vi "Z900_navX_I2C_Read.vi"(8 "error in (no error)":errorcluster, 10 "Registry":u8[](array[numeric]), 11 "Interface TypeDefs":T1 {"I2CDevRef"."Device Address" format="%.0x"}) -> (0 "error out":errorcluster, 1 "Valid":bool, 2 "Registry":u8[](array[numeric]), 3 "Interface TypeDefs":T1 {"I2CDevRef"."Device Address" format="%.0x"})   [LabVIEW 2015, in "navX Library v2.lvlib"]
uses:
  navX Library v2.lvlib
  TypeDefs/Z900_navX_InterfaceTypeDef.ctl
  <vilib>/Rock Robotics/WPI/SerialPort/WPI_SerialPortRef.ctl
  <vilib>/Rock Robotics/WPI/I2C/WPI_I2CDevRef.ctl
  <vilib>/Rock Robotics/SystemInterfaces/i2clib/i2c_bus.ctl
  <vilib>/Rock Robotics/WPI/SPI/WPI_SPIDevRef.ctl
  <vilib>/Rock Robotics/SystemInterfaces/spilib/spi_bus.ctl
  TypeDefs/Z900_navX_DeviceRegisters.ctl
  TypeDefs/Flags/Z900_navX_Flags_CapabilityTypeDef.ctl
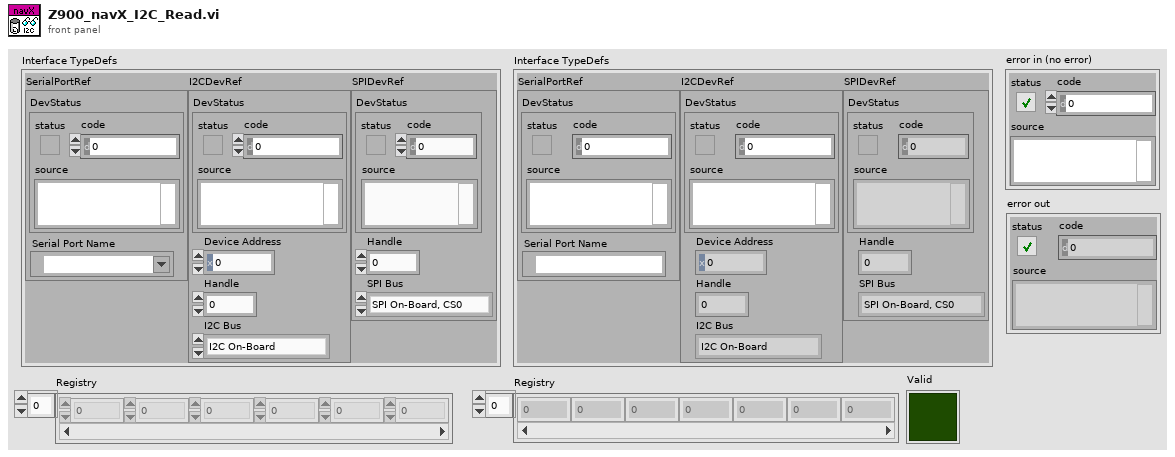
[diagram p1: front panel]
types:
  T1 = typedef "navX Library v2.lvlib/Z900_navX_InterfaceTypeDef.ctl" = cluster{"SerialPortRef":T2, "I2CDevRef":T3, "SPIDevRef":T5}
  T2 = typedef "WPI_SerialPortRef.ctl" = cluster{"DevStatus":errorcluster, "Serial Port Name":refnum<visa-resource-name>}
  T3 = typedef "WPI_I2CDevRef.ctl" = cluster{"DevStatus":errorcluster, "Device Address":u8, "Handle":i32, "I2C Bus":T4}
  T4 = typedef "i2c_bus.ctl" = enum16{"I2C On-Board", "I2C MXP", "Invalid"}
  T5 = typedef "WPI_SPIDevRef.ctl" = cluster{"DevStatus":errorcluster, "Handle":i32, "SPI Bus":T6}
  T6 = typedef "spi_bus.ctl" = enum16{"SPI On-Board, CS0", "SPI On-Board, CS1", "SPI On-Board, CS2", "SPI On-Board, CS3", "SPI MXP", "Invalid"}
  T7 = typedef "navX Library v2.lvlib/Z900_navX_DeviceRegisters.ctl" = u8
  T8 = typedef "navX Library v2.lvlib/Z900_navX_Flags_CapabilityTypeDef.ctl" = u16
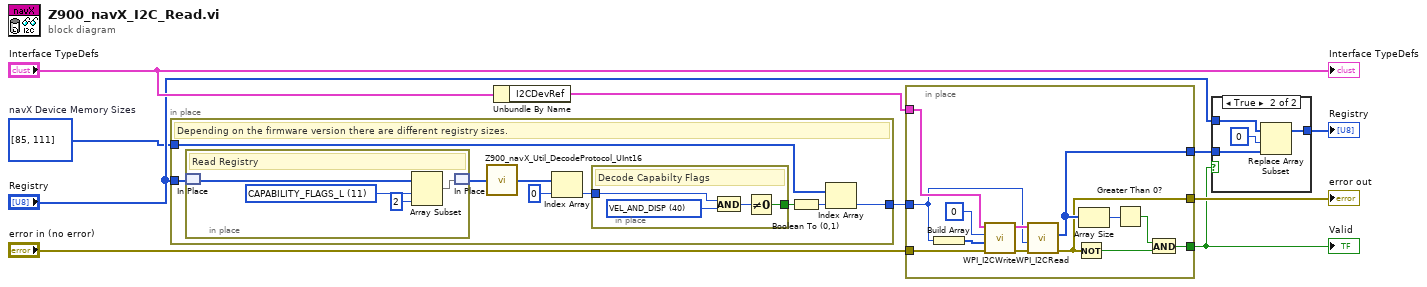
[diagram p0: block diagram]
diagram:
  w3 = i32[] [85, 111]  # navX Device Memory Sizes
  n1 = in-place {
    in-place-border: "Registry" -> [w19]
    in-place-border: w3 -> [w12]
    in-place-border: [w11] -> w8
    # "Depending on the firmware version there are different registry sizes."
    n2 = in-place {
      w27 = T7 11 items=["WHOAMI"=0, "HW_REV"=1, "FW_VER_MAJOR"=2, "FW_VER_MINOR"=3, "UPDATE_RATE_HZ"=4, "ACCEL_FSR_G"=5, "GYRO_FSR_DPS"=6, "OP_STATUS"=8, "CAL_STATUS"=9, "SELFTEST_STATUS"=10, "CAPABILITY_FLAGS_L"=11, "CAPABILITY_FLAGS_H"=12, "SENSOR_STATUS"=16, "TIMESTAMP"=18, "YAW"=22, "ROLL"=24, "PITCH"=26, "HEADING"=28, "FUSED_HEADING"=30, "ALTITUDE_I"=32, "ALTITUDE_D"=34, "LINERA_ACC_X"=36, "LINERA_ACC_Y"=38, "LINERA_ACC_Z"=40, "QUAT_W"=42, "QUAT_X"=44, "QUAT_Y"=46, "QUAT_Z"=48, "MPU_TEMP_C"=50, "GYRO_X"=52, "GYRO_Y"=54, "GYRO_Z"=56, "ACC_X"=58, "ACC_Y"=60, "ACC_Z"=62, "MAG_X"=64, "MAG_Y"=66, "MAG_Z"=68, "PRESSURE_I"=70, "PRESSURE_D"=72, "PRESSURE_TEMP"=74, "YAW_OFFSET"=76, "QUAT_OFFSET_W"=78, "QUAT_OFFSET_X"=80, "QUAT_OFFSET_Y"=82, "QUAT_OFFSET_Z"=84, "INTEGRATION_CONTROL"=86, "VELOCITY_X"=88, "VELOCITY_Y"=92, "VELOCITY_Z"=96, "DISPLACMENT_X"=100, "DISPLACMENT_Y"=104, "DISPLACEMENT_Z"=108] ("Device Register")
      # "Read Registry"
      n3 = in-place-match #1(w19) -> (w25:u8[])
      n4 = Array Subset(array=w25, index=w27, length=2) -> (w26:u8[])
      n5 = in-place-match #1(w26) -> (w16:u8[])
    }
    n6 = call "Z900_navX_Util_DecodeProtocol_UInt16.vi"("Little Endian"=w16) -> ("UInt16"=w17:u16[])
    n7 = Index Array(array=w17, index=0) -> (element=w15:u16)
    n8 = in-place {
      in-place-border: w15 -> [w21]
      in-place-border: [w20] -> w14
      w23 = T8 40 items=["OMNIMOUNT"=4, "OMNIMOUNT_CONFIG_MASK"=38, "VEL_AND_DISP"=40, "YAW_RESET"=80] ("Capability Flag")
      # "Decode Capabilty Flags"
      n9 = And(x=w21, y=w23) -> (x .and. y?=w22:T8)
      n10 = Not Equal To 0?(x=w22) -> (x != 0?=w20:bool)
    }
    n11 = Boolean To (0,1)(Boolean=w14) -> (0, 1=w13:i16)
    n12 = Index Array(array=w12, index=w13) -> (element=w11:i32)
  }
  n13 = Unbundle By Name("Interface TypeDefs") -> ("I2CDevRef"=w9:T3)
  n14 = in-place {
    in-place-border: [w34] -> w10
    in-place-border: [w33] -> w2
    in-place-border: w9 -> [w31]
    in-place-border: w8 -> [w30]
    in-place-border: [w29] -> w5
    in-place-border: "error in (no error)" -> [w28]
    n15 = Build Array(w30) -> (w40:i32[])
    n16 = call <vilib>:"WPI_I2CWrite.vi"("error in (no error)"=w28, "I2CDataToSend"=w40, "I2CRegister"=u8 0 ("hex"), "I2CDevRef"=w31) -> ("error out"=w39:errorcluster, "I2CDevRef"=w38:T3)  [unwired: 6 in]
    n17 = call <vilib>:"WPI_I2CRead.vi"("error in (no error)"=w39, "I2CBytesToRead"=w30, "I2CDevRef"=w38) -> ("error out"=w29:errorcluster, "Data Out"=w34:u8[])  [unwired: 6 in, 1 out]
    n18 = Not(x=w29) -> (.not. x?=w32:bool)
    n19 = Array Size(array=w34) -> (size(s)=w36:i32)
    n20 = Greater Than 0?(x=w36) -> (x > 0?=w35:bool)
    n21 = And(x=w35, y=w32) -> (x .and. y?=w33:bool)
  }
  "Valid" <- w2
  "error out" <- w5
  n22 = case shown="True" w2 {
    tunnel: "Registry" -> [w41 w45]
    tunnel: [w41 w44] -> w1
    tunnel: w10 -> [_ w43]
    frame False {
    }
    frame True {
      n23 = Replace Array Subset(array=w45, new element=w43, index=u8 0 ("hex")) -> (w44:u8[])
    }
  }
  "Registry" <- w1
  "Interface TypeDefs" <- "Interface TypeDefs"
